vi "事件结构.vi"() -> ()   [LabVIEW 2017]
panel:
  out "字符串":string
  in  "close":bool
  in  "open":bool
  out "light":bool
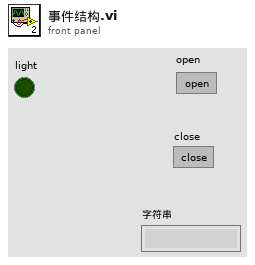
[diagram p1: front panel]
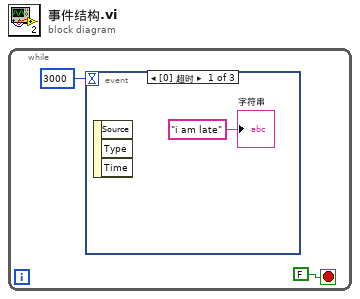
[diagram p0: block diagram]
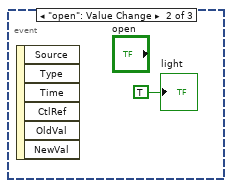
[diagram p2: hidden frame]
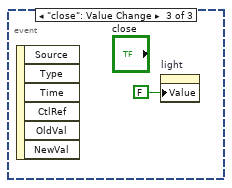
[diagram p3: hidden frame]
diagram:
  n1 = while {
    stop <- FALSE stop-if-true
    n2 = event shown="[0] 超时" {
      selector: _ -> [_ _ _]
      dyn-events: _ -> [_ _ _]
      timeout: 3000 -> [_ _ _]
      event Timeout {
        n3 = event-data() -> ()  [unwired: 1 in, 3 out]
        "字符串" <- "i am late" ("字符串")
      }
      event "open": Value Change {
        n4 = event-data() -> ()  [unwired: 1 in, 6 out]
        "light" <- TRUE ("light")
      }
      event "close": Value Change {
        n5 = event-data() -> ()  [unwired: 1 in, 6 out]
        n6 = property on="light" class="Bool (严格)"("Value"=FALSE ("light")) -> ()  [unwired: 2 in, 2 out]
      }
    }
  }
